vi "Check.vi"(8 "error in (no error)":errorcluster, 11 "Protocol in":refnum<class "Protocol.lvclass">) -> (0 "error out":errorcluster, 2 "Still alive?":bool, 3 "Protocol out":refnum<class "Protocol.lvclass">)   [LabVIEW 2017, in "FileSync -- Base.lvlib" / "Protocol.lvclass"]
uses:
  Protocol.lvclass
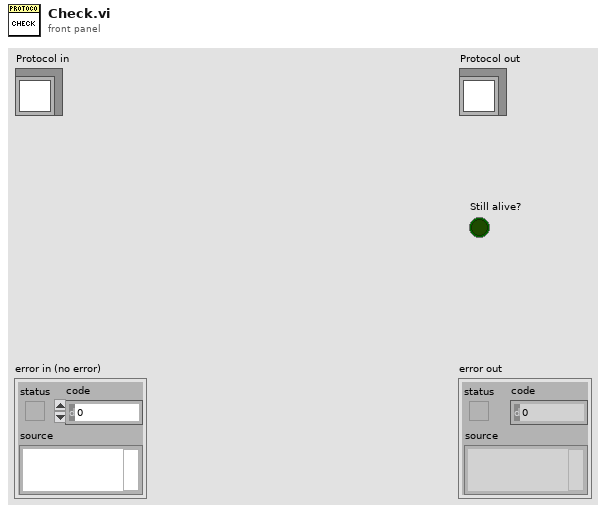
[diagram p1: front panel]
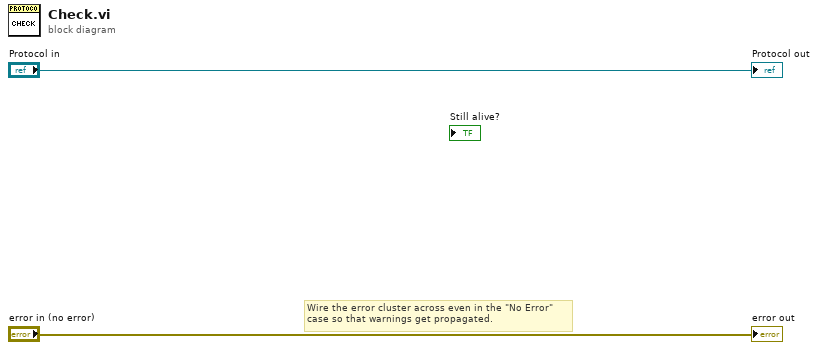
[diagram p0: block diagram]
diagram:
  # "Wire the error cluster across even in the \"No Error\"\ncase so that warnings get propagated."
  "error out" <- "error in (no error)"
  "Protocol out" <- "Protocol in"
